vi "Send FPGA Responses.vi"(8 "error in (no error)":errorcluster, 11 "Data":variant) -> (0 "error out":errorcluster)   [LabVIEW 2023, in "Encoder.lvlib"]
uses:
  Encoder.lvlib
  Internal Communication/Controls/Base Message.ctl
  Internal Communication/Internal Communication.lvlib
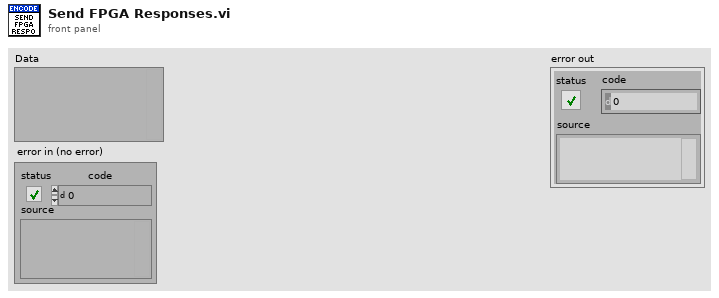
[diagram p1: front panel]
types:
  T1 = typedef "Internal Communication.lvlib/Base Message.ctl" = cluster{"Command":string, "Data":variant}
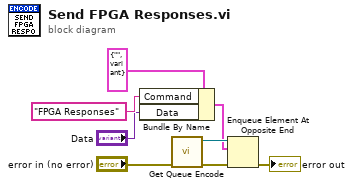
[diagram p0: block diagram]
diagram:
  n1 = Bundle By Name(cluster=T1 {"Command"="", "Data"=variant} ("Message"), "Command"="FPGA Responses", "Data"="Data") -> (w6:T1)
  n2 = call "Get Queue Encode.vi"("error in (no error)"="error in (no error)") -> ("error out"=w8:errorcluster, "Decoder Queue"=w7:refnum<queue>)  [unwired: 9 in]
  n3 = Enqueue Element At Opposite End(queue=w7, element=w6, error in (no error)=w8) -> (error out=→"error out":errorcluster)  [unwired: 1 in, 2 out]
